vi "GetValueType.vi"(0 "variant":variant, 11 "error in":errorcluster) -> (4 "variant out":variant, 6 "Value Type":T1, 15 "error out":errorcluster)   [LabVIEW 2019]
uses:
  Valuetype.ctl
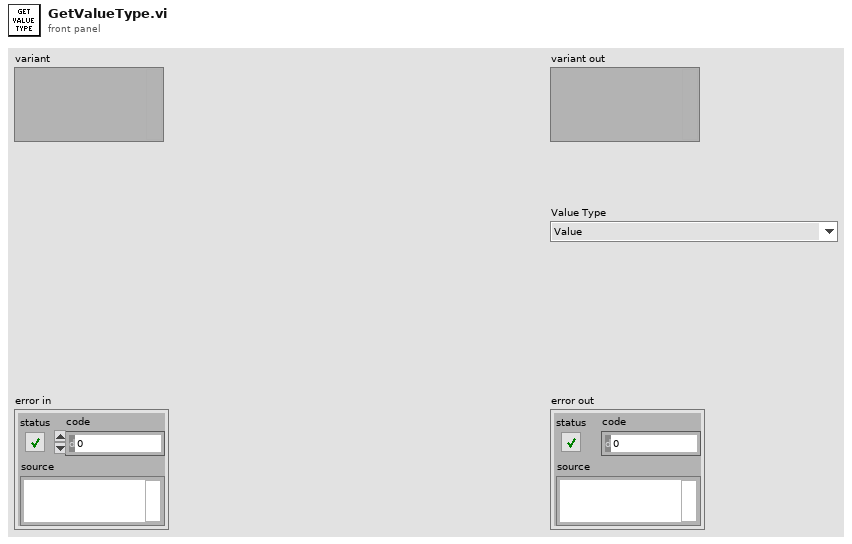
[diagram p1: front panel]
types:
  T1 = typedef "Valuetype.ctl" = enum16{"Value", "Variable", "Function"}
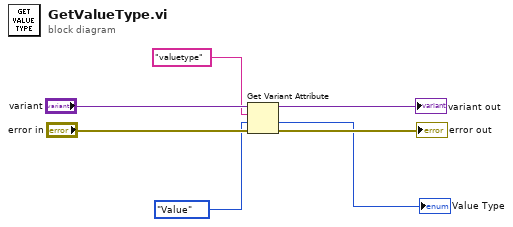
[diagram p0: block diagram]
diagram:
  n1 = Get Variant Attribute(Variant="variant", name="valuetype", default value (empty Variant)=Valuetype."Value" ("valuetype"), error in="error in") -> (duplicate Variant=→"variant out":variant, value=→"Value Type":T1, error out=→"error out":errorcluster)  [unwired: 1 out]
